vi "pracTimeInRange.vi"() -> ()   [LabVIEW 2020]
uses:
  Control 1.ctl
panel:
  out "Enum":T1
  in  "Y":dbl
  in  "X":dbl
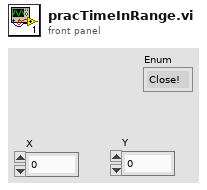
[diagram p1: front panel]
types:
  T1 = typedef "Control 1.ctl" = enum16{"Close!", "Almost There!", "Good!", "Great!"}
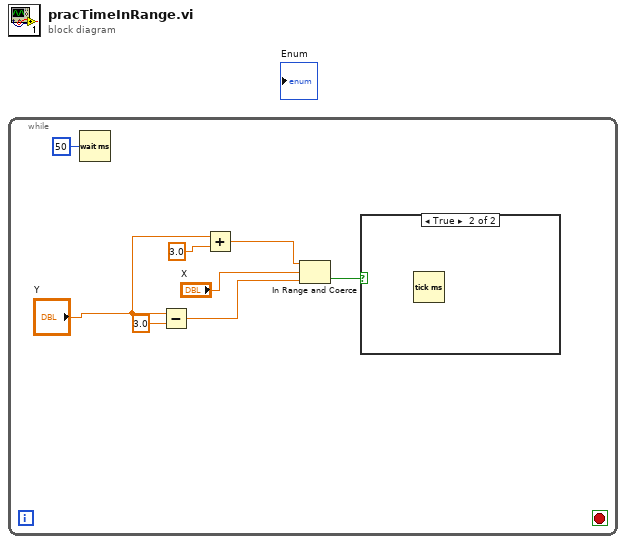
[diagram p0: block diagram]
diagram:
  n1 = while {
    stop <- _ stop-if-true
    n2 = Wait (ms)(milliseconds to wait=u32 50) -> ()  [unwired: 1 out]
    n3 = Subtract(x="Y", y=3.0) -> (x-y=w6:dbl)
    n4 = Add(x="Y", y=3.0) -> (x+y=w2:dbl)
    n5 = In Range and Coerce(upper limit=w2, x="X", lower limit=w6) -> (In Range?=w1:bool)  [unwired: 1 out]
    n6 = case shown="True" w1 {
      frame False {
      }
      frame True {
        n7 = Tick Count (ms)() -> ()  [unwired: 1 out]
      }
    }
  }
